vi "1. 主程序：输入 + 显示.vi"() -> ()   [LabVIEW 2018]
panel:
  in  ">1000 数据点 红色":u32(colorbox)=13107200
  in  "<1000 数据点 橘色":u32(colorbox)=16732970
  in  "<400 数据点 黄色":u32(colorbox)=16769858
  in  "<120 数据点 灰色":u32(colorbox)=11121611
  in  "<-120 数据点 青色":u32(colorbox)=2817023
  in  "<-300 数据点 蓝色":u32(colorbox)=16777224
  out "显示；管道+光纤+数据 分布":picture
  in  "数据文件名":string="1_第1个设计的data.txt"
  in  "选择：光纤后段 颜色":u32(colorbox)=14780529 caption="选择：光纤 - 后段 颜色"
  out "显示：管道 分布":picture
  out "显示：管道+光纤 分布":picture caption="显示；管道+光纤 分布"
  in  "输入：放大倍数":i32=30
  in  "选择：管道 颜色":u32(colorbox)=8816506 caption="选择：管道颜色"
  in  "选择：光纤前段 颜色":u32(colorbox)=6927784 caption="选择：光纤 - 前段 颜色"
  in  "输入：平移图像":dbl[](array[numeric])=[0.0, 0.0]
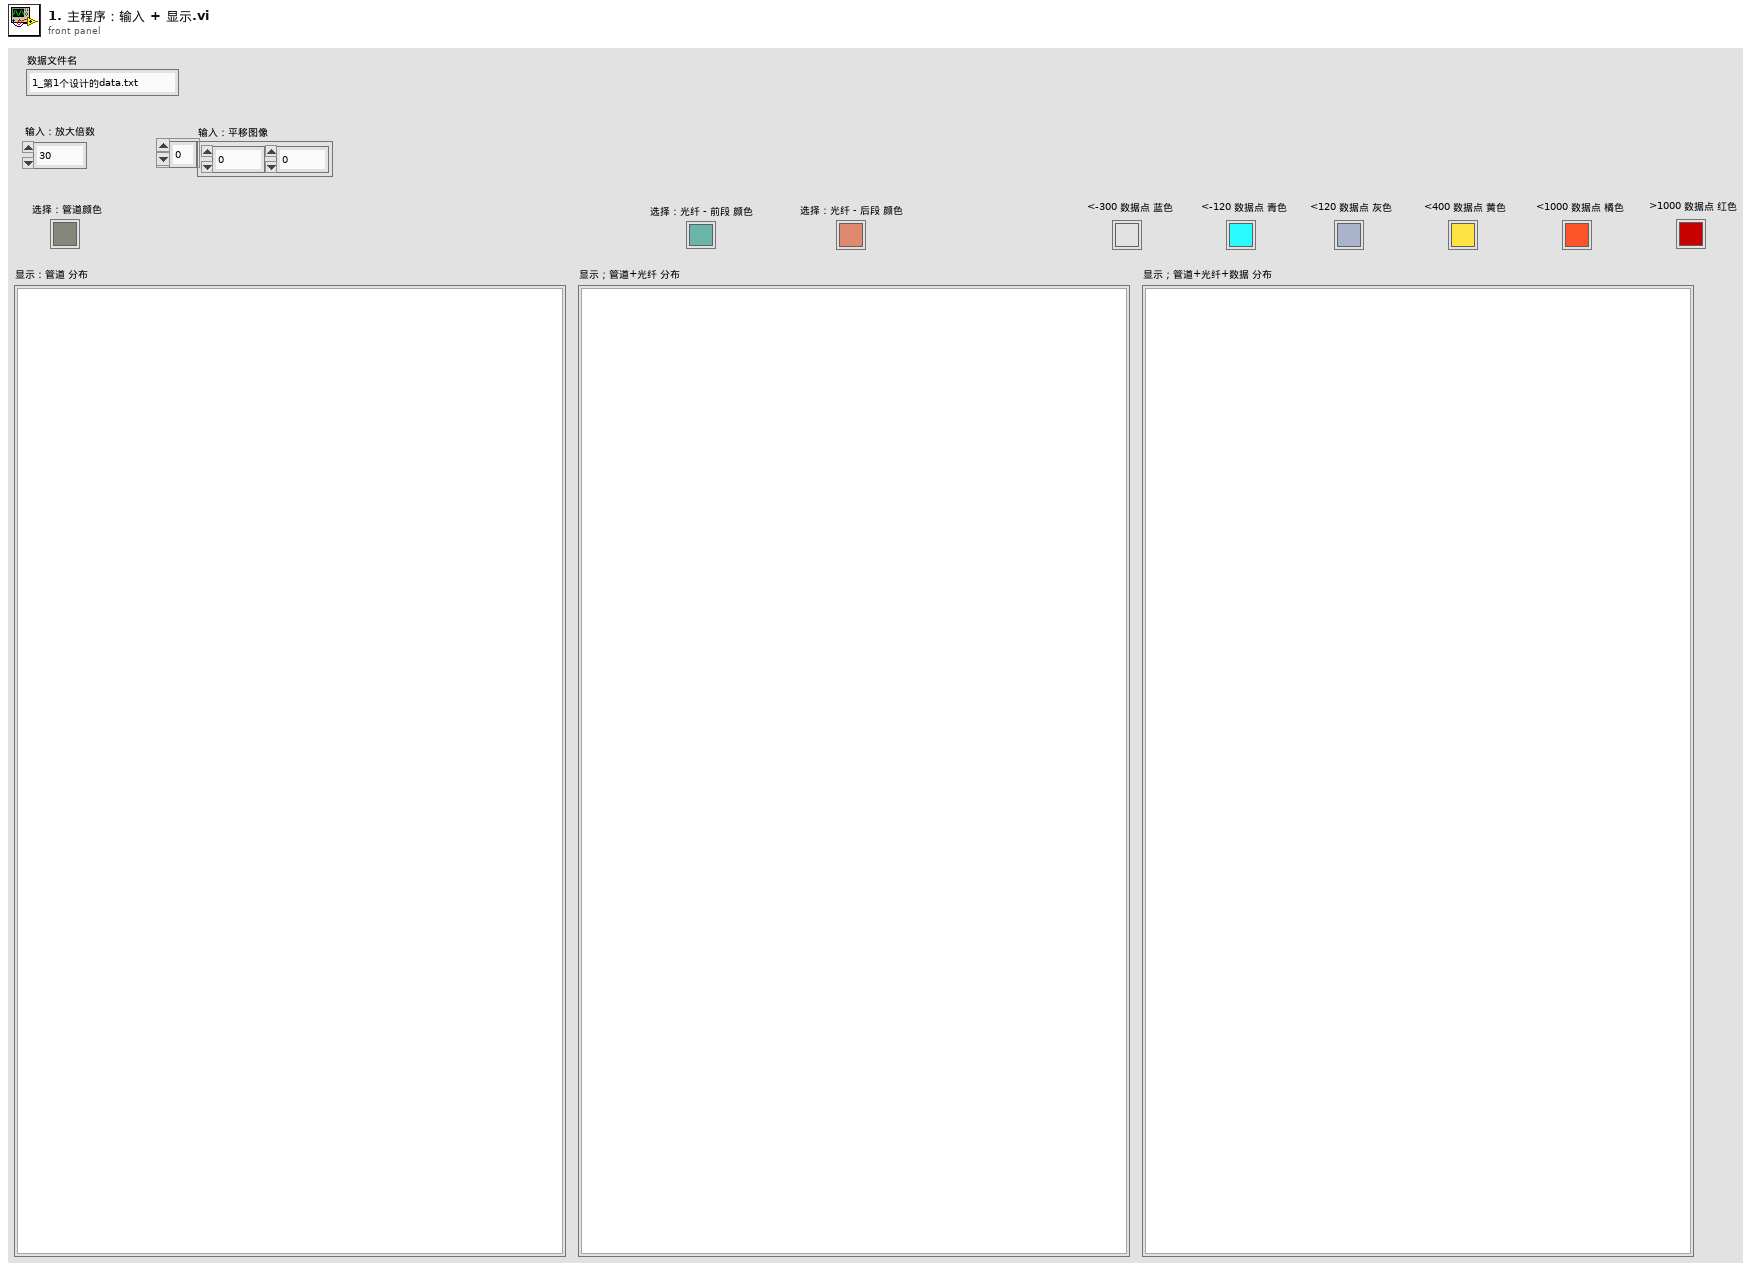
[diagram p1: front panel]
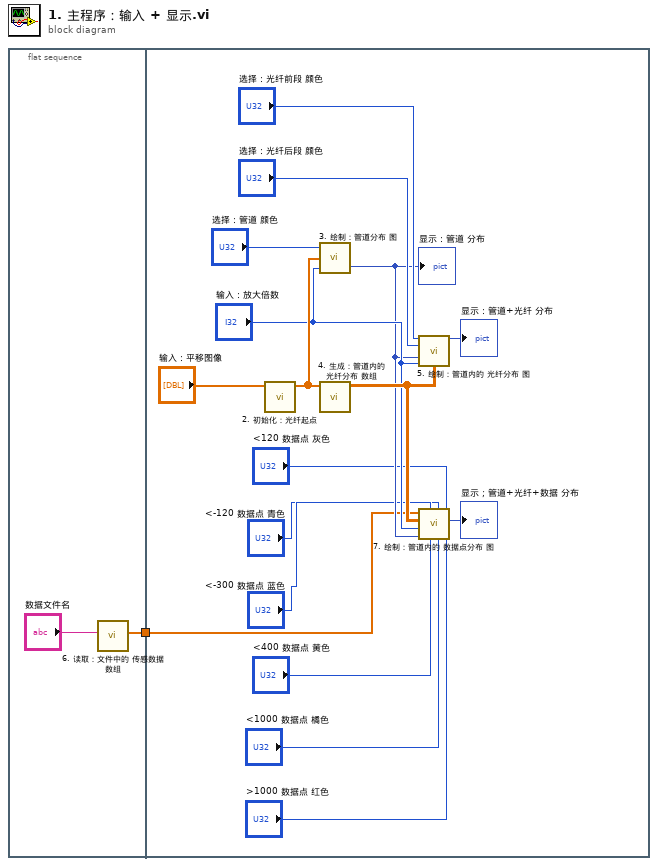
[diagram p0: block diagram]
diagram:
  n1 = flat-sequence {
    tunnel: [w2] -> w1
    tunnel: w1 -> [w4]
    frame #0 {
      n2 = call "6. 读取：文件中的 传感数据 数组.vi"("数据文件名"="数据文件名") -> ("解析出的 浮点数据"=w2:dbl[])  [unwired: 8 in, 1 out]
    }
    frame #1 {
      n3 = call "2. 初始化：光纤起点.vi"("初始偏移量：相对于起点(14,27)"="输入：平移图像") -> ("坐标原点 重新选定后 的 一维数组"=w15:dbl[])  [unwired: 10 in]
      n4 = call "3. 绘制：管道分布 图.vi"("放大倍数"="输入：放大倍数", "坐标原点 重新选定后 的 一维数组"=w15, "color(black)输入"="选择：管道 颜色") -> ("管道分布"=w12:picture)  [unwired: 1 in]
      "显示：管道 分布" <- w12
      n5 = call "4. 生成：管道内的 光纤分布 数组.vi"("光纤起点"=w15) -> ("光纤分布"=w14:dbl[][])  [unwired: 9 in]
      n6 = call "5. 绘制：管道内的 光纤分布 图.vi"("光纤：前段 颜色"="选择：光纤前段 颜色", "光纤：后段 颜色"="选择：光纤后段 颜色", "管道分布"=w12, "输入：放大"="输入：放大倍数", "光纤分布"=w14) -> ("显示：管道+光纤分布"=→"显示：管道+光纤 分布":picture)  [unwired: 10 in]
      n7 = call "7. 绘制：管道内的 数据点分布 图.vi"(">1000 数据点 红色"=">1000 数据点 红色", "<120 数据点 灰色"="<120 数据点 灰色", "<1000 数据点 橘色"="<1000 数据点 橘色", "<-120 数据点 青色"="<-120 数据点 青色", "<400 数据点 黄色"="<400 数据点 黄色", "<-300 数据点 蓝色"="<-300 数据点 蓝色", "管道分布"=w12, "输入：放大倍数"="输入：放大倍数", "光纤分布"=w14, "数据分布 一维数组"=w4) -> ("管道+数据分布"=→"显示；管道+光纤+数据 分布":picture)  [unwired: 1 in]
    }
  }
